vi "Example_Simple_Set_Get Functios_StringFormat.vi"() -> ()   [LabVIEW 2020]
doc: "Demonstrates how GUI object values can be converted into string values. The multiple controls can be accessed using just single user event case."
uses:
  VI Server Libraries/VI Server_Set Controls.llb/Set STR Control.vi
  VI Server Toolkit LV2013.lvlib
panel:
  in  "Tab.Main":enum32{"Set/Get1", "Set/Get2"}(tab)
  in  "CtlValue.String":string caption="Control Value: String"
  in  "File Path.Mirror":path
  in  "Numeric.Mirror":dbl=5.0 caption="Numeric Control"
  in  "Slide.Mirror":dbl(slide)=1.9191919191919191 caption="Horizontal Fill Slide" scale=0.0..10.0
  in  "Knob.Mirror":dbl(knob) caption="Knob" scale=0.0..10.0
  in  "Button.Mirror":bool caption="Settings Button"
  in  "Menu Ring.Mirror":u16(ring) caption="Menu Ring" items=["Item 1", "Item 2", "Item 3"]
  in  "LED.Mirror":bool caption="LED"
  in  "1D Array - String.Mirror":string[](array[string]) caption="1D Array - String"
  in  "2D Array - String.Mirror":string[][](array[string]) caption="2D Array - String"
  in  "1D Array - DBL.Mirror":dbl[](array[numeric]) caption="1D Array - DBL"
  in  "2D Array - DBL.Mirror":dbl[][](array[numeric]) caption="2D Array - DBL"
  in  "2D Array - Path.Mirror":path[][](array[path]) caption="2D Array - String"
  in  "2D Array - Boolean.Mirror":bool[][](array[boolean]) caption="2D Array - String"
  in  "ArrayCtlValue.String":string caption="Control Value: String"
  in  "EXIT":bool
  in  "Error In":errorcluster
  out "error out":errorcluster
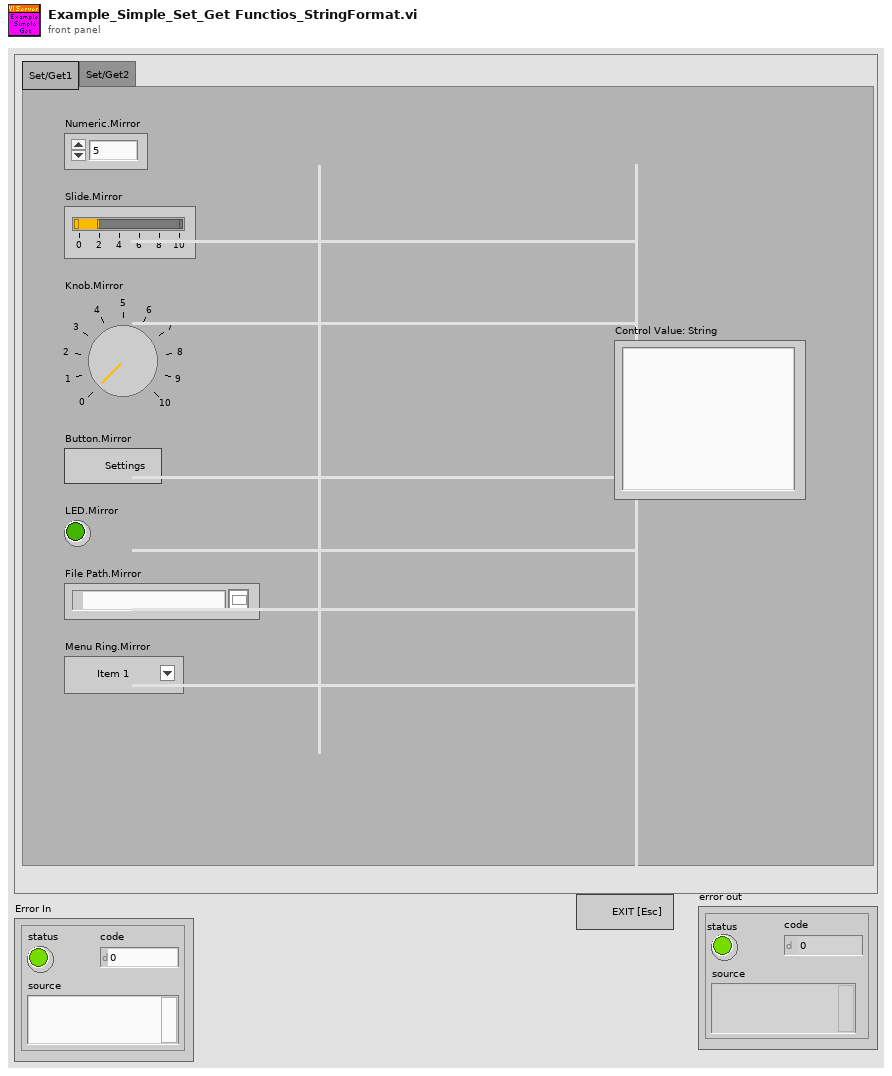
[diagram p1: front panel]
types:
  T1 = typedef "VI Server_RefsCluster.ctl" = cluster{"Labels":string[], "Refs":refnum<vi>[], "VI Ref":refnum<vi>}
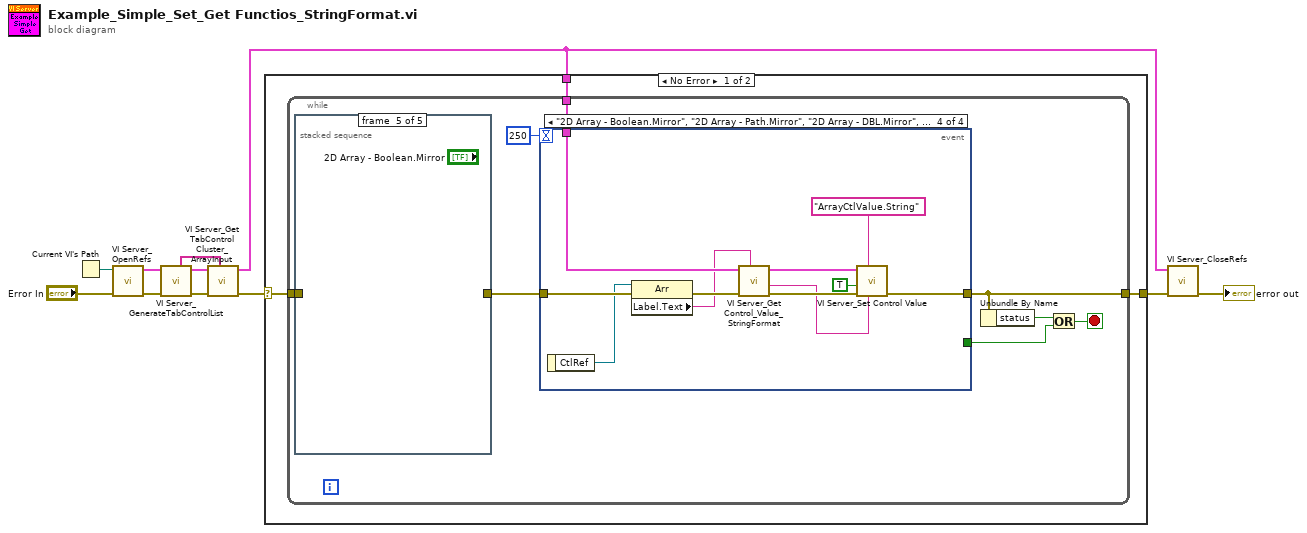
[diagram p0: block diagram]
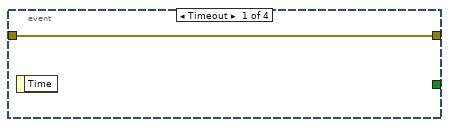
[diagram p2: hidden frame]
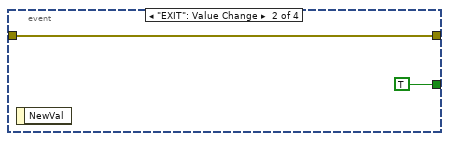
[diagram p3: hidden frame]
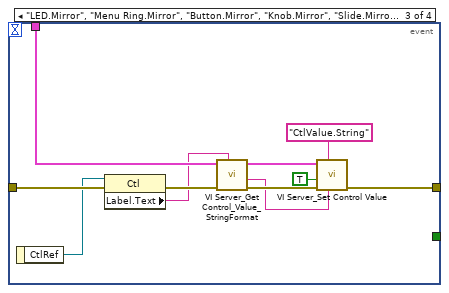
[diagram p4: hidden frame]
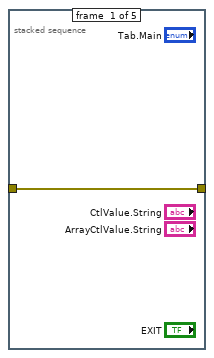
[diagram p5: hidden frame]
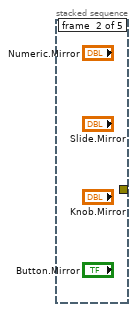
[diagram p6: hidden frame]
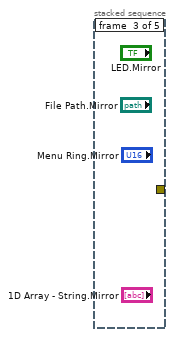
[diagram p7: hidden frame]
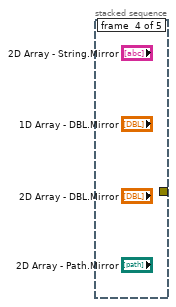
[diagram p8: hidden frame]
diagram:
  n1 = Current VI's Path() -> (path=w10:path)
  n2 = call "VI Server_OpenRefs.vi"("error in"="Error In", "VI Path"=w10) -> ("error out"=w4:errorcluster, "VI Server.RefsCluster"=w5:T1)  [unwired: 8 in]
  n3 = call "VI Server_GenerateTabControlList.vi"("error in (no error)"=w4, "VI Server Cluster"=w5) -> ("error out"=w7:errorcluster, "VI Server Cluster.DUP"=w6:T1, "TabControls"=w2:string[])  [unwired: 7 in]
  n4 = call "VI Server_Get TabControl Cluster_ArrayInput.vi"("TabControl Labels[]"=w2, "error in"=w7, "VI Server Cluster"=w6) -> ("error out"=w3:errorcluster, "VI Server Cluster.OUT"=w1:T1)  [unwired: 7 in]
  n5 = case shown="No Error" w3 {
    selector: w3 -> [w14 w49]
    tunnel: [w13 w49] -> w9
    tunnel: w1 -> [w12 _]
    frame No Error {
      n6 = while {
        tunnel: w14 -> [w21]
        tunnel: [w19] -> w13
        tunnel: w12 -> [w15]
        stop <- w16 stop-if-true
        n7 = stacked-sequence {
          tunnel: [w48 _ _ _ _] -> w20
          tunnel: w21 -> [w48 _ _ _ _]
          frame #0 {
          }
          frame #1 {
          }
          frame #2 {
          }
          frame #3 {
          }
          frame #4 {
          }
        }
        n8 = event shown="[3] \"2D Array - Boolean.Mirror\", \"2D Array - Path.Mirror\", \"2D Array - DBL.Mirror\", \"1D Array - DBL.Mirror\", \"2D Array - String.Mirror\", \"1D Array - String.Mirror\": Value Change" {
          selector: _ -> [_ _ _ _]
          dyn-events: _ -> [_ _ _ _]
          timeout: 250 -> [_ _ _ _]
          tunnel: w20 -> [w23 w25 w29 w40]
          tunnel: [w23 w25 w36 w43] -> w19
          tunnel: [_ TRUE _ _] -> w17
          tunnel: w15 -> [_ _ w32 w47]
          event Timeout {
            n9 = event-data() -> ()  [unwired: 1 in, 1 out]
          }
          event "EXIT": Value Change {
            n10 = event-data() -> ()  [unwired: 1 in, 1 out]
          }
          event "LED.Mirror", "Menu Ring.Mirror", "Button.Mirror", "Knob.Mirror", "Slide.Mirror", "Numeric.Mirror", "File Path.Mirror": Value Change {
            n11 = event-data() -> ("CtlRef"=w27:refnum<vi>)  [unwired: 1 in]
            n12 = property class="Ctl"(reference=w27, error in=w29) -> (error out=w28:errorcluster, "Label.Text"=w26:string)  [unwired: 1 out]
            n13 = call "VI Server_Get Control_Value_StringFormat.vi"("Label"=w26, "error in (no error)"=w28, "VI Server Cluster"=w32) -> ("error out"=w33:errorcluster, "ControlValue(StringFormat)"=w31:string, "VI Server Cluster.DUP"=w30:T1)  [unwired: 5 in, 1 out]
            n14 = call-poly "VI Server_Set Control Value.vi"("New Value"=w31, "Label"="CtlValue.String", "error in"=w33, "Single Instance (T)"=TRUE, "VI Server Cluster"=w30) -> ("error out"=w36:errorcluster)  [unwired: 4 in, 2 out]
          }
          event "2D Array - Boolean.Mirror", "2D Array - Path.Mirror", "2D Array - DBL.Mirror", "1D Array - DBL.Mirror", "2D Array - String.Mirror", "1D Array - String.Mirror": Value Change {
            n15 = event-data() -> ("CtlRef"=w38:refnum<vi>)  [unwired: 1 in]
            n16 = property class="Arr"(reference=w38, error in=w40) -> (error out=w39:errorcluster, "Label.Text"=w37:string)  [unwired: 1 out]
            n17 = call "VI Server_Get Control_Value_StringFormat.vi"("Label"=w37, "error in (no error)"=w39, "VI Server Cluster"=w47) -> ("error out"=w46:errorcluster, "ControlValue(StringFormat)"=w41:string, "VI Server Cluster.DUP"=w45:T1)  [unwired: 5 in, 1 out]
            n18 = call-poly "VI Server_Set Control Value.vi"("New Value"=w41, "Label"="ArrayCtlValue.String", "error in"=w46, "Single Instance (T)"=TRUE, "VI Server Cluster"=w45) -> ("error out"=w43:errorcluster)  [unwired: 4 in, 2 out]
          }
        }
        n19 = Unbundle By Name(w19) -> ("status"=w18:bool)
        n20 = Or(x=w18, y=w17) -> (x .or. y?=w16:bool)
      }
    }
    frame Error {
    }
  }
  n21 = call "VI Server_CloseRefs.vi"("error in"=w9, "VI Server.RefsCluster"=w1) -> ("error out"=→"error out":errorcluster)  [unwired: 9 in]
